vi "create_AnalysisObject.vi"(8 "error in (no error)":errorcluster, 10 "FilePath":path) -> (0 "error out":errorcluster, 3 "Analysis out":refnum<class "Analysis.lvclass">)   [LabVIEW 2015]
doc: "loads the data from the file path and creates an AnalysisObject that stores all the data of this analysis.\nThe VI returns the AnalysisObject"
uses:
  MSControl/Classes/Analysis/Analysis.lvclass
  MSControl/Classes/DataLoggingText/DataLogging.lvclass
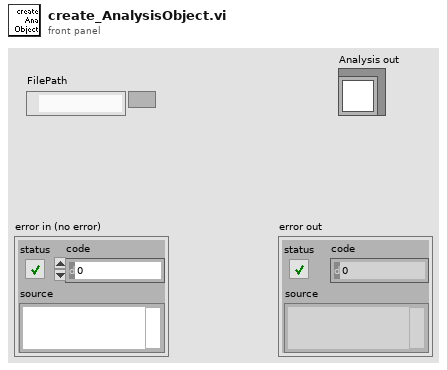
[diagram p1: front panel]
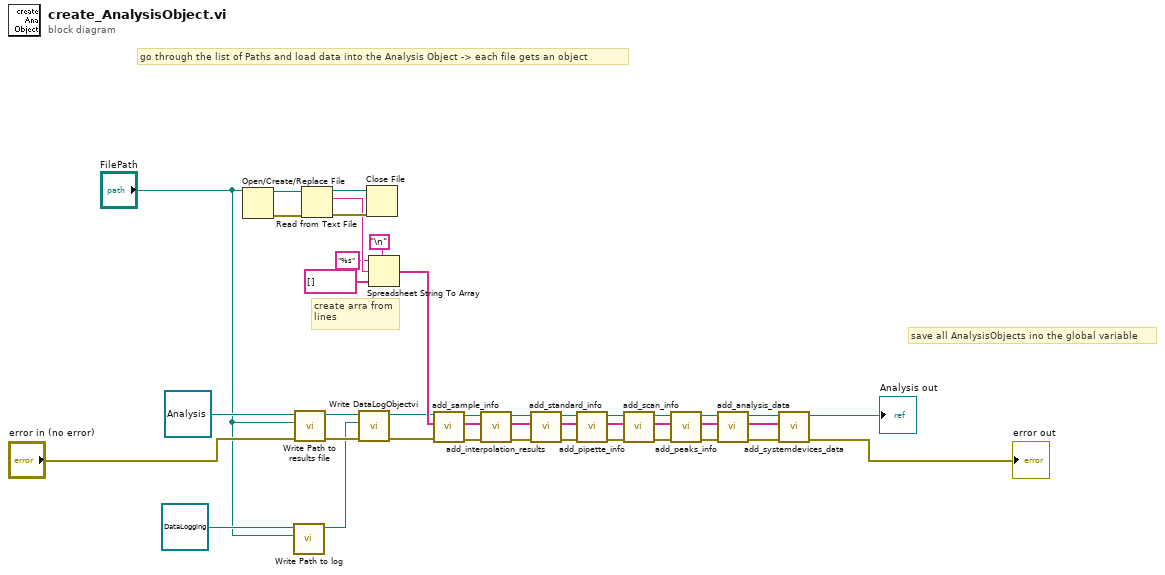
[diagram p0: block diagram]
diagram:
  # "create arra from\nlines"
  # "save all AnalysisObjects ino the global variable"
  # "go through the list of Paths and load data into the Analysis Object -> each file gets an object"
  n1 = Open/Create/Replace File(file path (use dialog)="FilePath") -> (refnum out=w40:refnum<file>, error out=w39:errorcluster)  [unwired: 5 in, 1 out]
  n2 = call-dynamic "Write Path to log.vi"("Path to log"="FilePath", "DataLoggingText in"=refnum<class "DataLogging.lvclass"> refnum ("DataLoggingText.lvclass")) -> ("DataLoggingText out"=w7:refnum<class "DataLogging.lvclass">)  [unwired: 8 in, 1 out]
  n3 = call-dynamic "Write Path to results file.vi"("error in (no error)"="error in (no error)", "Path to results file"="FilePath", "Analysis in"=refnum<class "Analysis.lvclass"> refnum ("Analysis.lvclass")) -> ("error out"=w9:errorcluster, "Analysis out"=w11:refnum<class "Analysis.lvclass">)  [unwired: 7 in]
  n4 = Read from Text File(file (use dialog)=w40, error in=w39) -> (refnum out=w38:refnum<file>, text=w35:string, error out=w37:errorcluster)  [unwired: 2 in, 1 out]
  n5 = call-dynamic "Write DataLogObjectvi.vi"("error in (no error)"=w9, "DataLogging.lvclass"=w7, "Analysis in"=w11) -> ("error out"=w8:errorcluster, "Analysis out"=w10:refnum<class "Analysis.lvclass">)  [unwired: 7 in]
  n6 = Close File(refnum=w38, error in=w37) -> ()  [unwired: 2 out]
  n7 = Spreadsheet String To Array(delimiter (Tab)="\n", format string="%s", spreadsheet string=w35, array type (2D Dbl)=string[] []) -> (array=w31:string[])
  n8 = call "add_sample_info.vi"("error in (no error)"=w8, "data array"=w31, "Analysis in"=w10) -> ("error out"=w29:errorcluster, "data array out"=w28:string[], "Analysis out"=w30:refnum<class "Analysis.lvclass">)  [unwired: 6 in]
  n9 = call "add_interpolation_results.vi"("error in (no error)"=w29, "data array"=w28, "Analysis in"=w30) -> ("error out"=w26:errorcluster, "data array out"=w25:string[], "Analysis out"=w27:refnum<class "Analysis.lvclass">)  [unwired: 6 in]
  n10 = call "add_standard_info.vi"("error in (no error)"=w26, "data array"=w25, "Analysis in"=w27) -> ("error out"=w22:errorcluster, "data array out"=w23:string[], "Analysis out"=w24:refnum<class "Analysis.lvclass">)  [unwired: 6 in]
  n11 = call "add_pipette_info.vi"("error in (no error)"=w22, "data array"=w23, "Analysis in"=w24) -> ("error out"=w20:errorcluster, "data array out"=w19:string[], "Analysis out"=w21:refnum<class "Analysis.lvclass">)  [unwired: 6 in]
  n12 = call "add_scan_info.vi"("error in (no error)"=w20, "data array"=w19, "Analysis in"=w21) -> ("error out"=w17:errorcluster, "data array out"=w16:string[], "Analysis out"=w18:refnum<class "Analysis.lvclass">)  [unwired: 6 in]
  n13 = call "add_peaks_info.vi"("error in (no error)"=w17, "data array"=w16, "Analysis in"=w18) -> ("error out"=w14:errorcluster, "data array out"=w13:string[], "Analysis out"=w15:refnum<class "Analysis.lvclass">)  [unwired: 6 in]
  n14 = call "add_analysis_data.vi"("error in (no error)"=w14, "data array"=w13, "Analysis in"=w15) -> ("error out"=w4:errorcluster, "data array out"=w1:string[], "Analysis out"=w5:refnum<class "Analysis.lvclass">)  [unwired: 6 in]
  n15 = call "add_systemdevices_data.vi"("error in (no error)"=w4, "data array"=w1, "Analysis in"=w5) -> ("error out"=→"error out":errorcluster, "Analysis out"=→"Analysis out":refnum<class "Analysis.lvclass">)  [unwired: 6 in, 1 out]
